vi "Write Power.vi"(8 "error in (no error)":errorcluster, 9 "Right Power":dbl(slide)=1.0 min=-1.0 max=1.0 step=0.01 scale=-1.0..1.0, 10 "Left Power":dbl(slide)=1.0 min=-1.0 max=1.0 step=0.01 scale=-1.0..1.0, 11 "Drive by Power in":refnum<class "Drive by Power.lvclass">) -> (0 "error out":errorcluster, 3 "Drive by Power out":refnum<class "Drive by Power.lvclass">)   [LabVIEW 2013, in "Logical Systems.lvlib" / "Drive Train.lvlib" / "Drive by Power.lvlib" / "Drive by Power.lvclass"]
uses:
  Drive by Power.lvclass
  Drive by Power.lvclass/Drive by Power.ctl
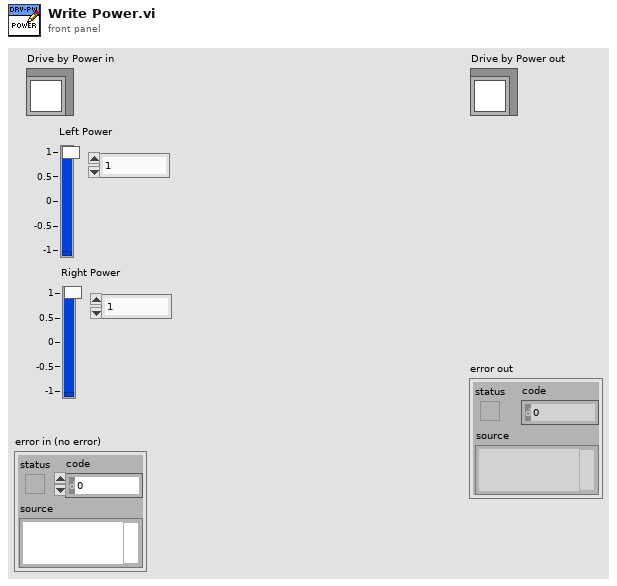
[diagram p1: front panel]
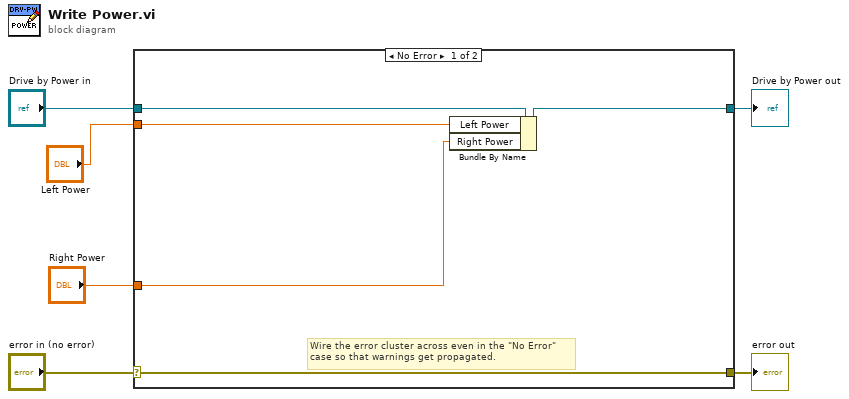
[diagram p0: block diagram]
diagram:
  n1 = case shown="No Error" "error in (no error)" {
    selector: "error in (no error)" -> [w10 w13]
    tunnel: [w10 w13] -> w5
    tunnel: [w9 w12] -> w3
    tunnel: "Drive by Power in" -> [w11 w12]
    tunnel: "Left Power" -> [w8 _]
    tunnel: "Right Power" -> [w7 _]
    frame No Error {
      # "Wire the error cluster across even in the \"No Error\"\ncase so that warnings get propagated."
      n2 = Bundle By Name(cluster=w11, "Left Power"=w8, "Right Power"=w7) -> (w9:refnum<class "Drive by Power.lvclass">)
    }
    frame Error {
    }
  }
  "error out" <- w5
  "Drive by Power out" <- w3
